vi "TestForceGraph 1.vi"() -> ()   [LabVIEW 2017]
panel:
  out "Signal Up":T1
  in  "FirstTouchAuto":T2={"FirstPeakforce"=2.0, "F_LengthView"=20, "A_LengthView "=10}
  in  "Auto":bool
  in  "FirstTouchDown":T2={"FirstPeakforce"=3.0, "F_LengthView"=20, "A_LengthView "=15}
  in  "ShowName":cluster{"ShowArrow":bool, "Alias":bool}
  in  "AngleMaxForce":bool=TRUE
  out "XY Up":cluster{"Y":dbl[], "Y":dbl[]}[](graph)
  in  "First Touch":bool
  in  "Path":path
  out "Filenames":string[](array[string])
  in  "FileType":string(combo)="DL"
  out "XY Down":cluster{"Y":dbl[], "Y":dbl[]}[](graph)
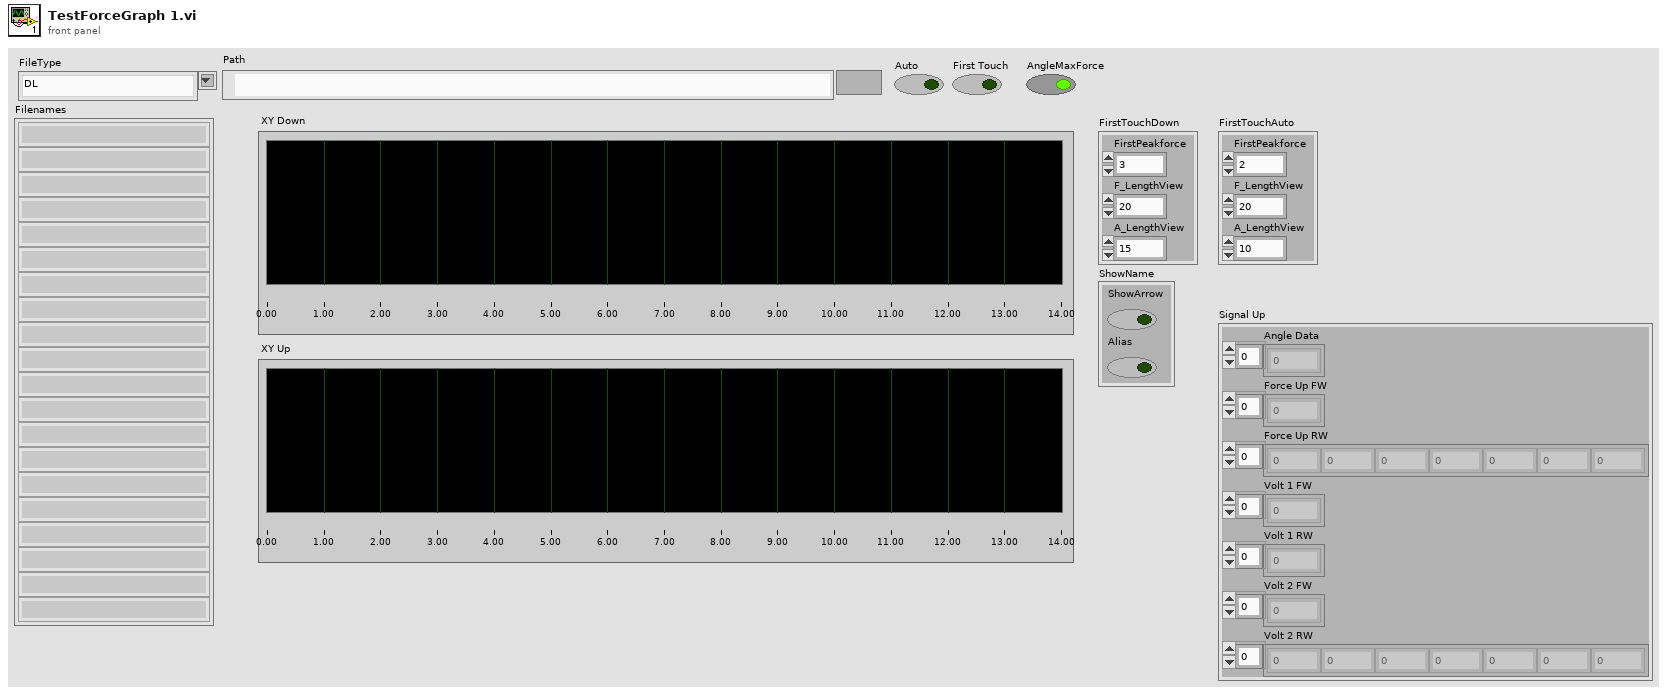
[diagram p1: front panel]
types:
  T1 = cluster{"Angle Data":dbl[], "Force Up FW":dbl[], "Force Up RW":dbl[], "Volt 1 FW":dbl[], "Volt 1 RW":dbl[], "Volt 2 FW":dbl[], "Volt 2 RW":dbl[]}
  T2 = cluster{"FirstPeakforce":dbl, "F_LengthView":i32, "A_LengthView ":i32}
  T3 = cluster{"DownMax":u16, "DownMin":u16, "UpMax":u16, "UpMin":u16}
  T4 = cluster{"Peak_Force":dbl, "Peak_Force_Tolerance":dbl, "Full_Angle":dbl, "Full_Angle_Tolerance":dbl, "ReturnForce":dbl}
  T5 = cluster{"Angle Data":dbl[], "Force Data":dbl[], "Volt Data 1":dbl[], "Volt Data 2":dbl[]}
  T6 = cluster{"Angle Data":dbl[], "Force Down FW":dbl[], "Force Down RW":dbl[], "Volt 1 FW":dbl[], "Volt 1 RW":dbl[], "Volt 2 FW":dbl[], "Volt 2 RW":dbl[]}
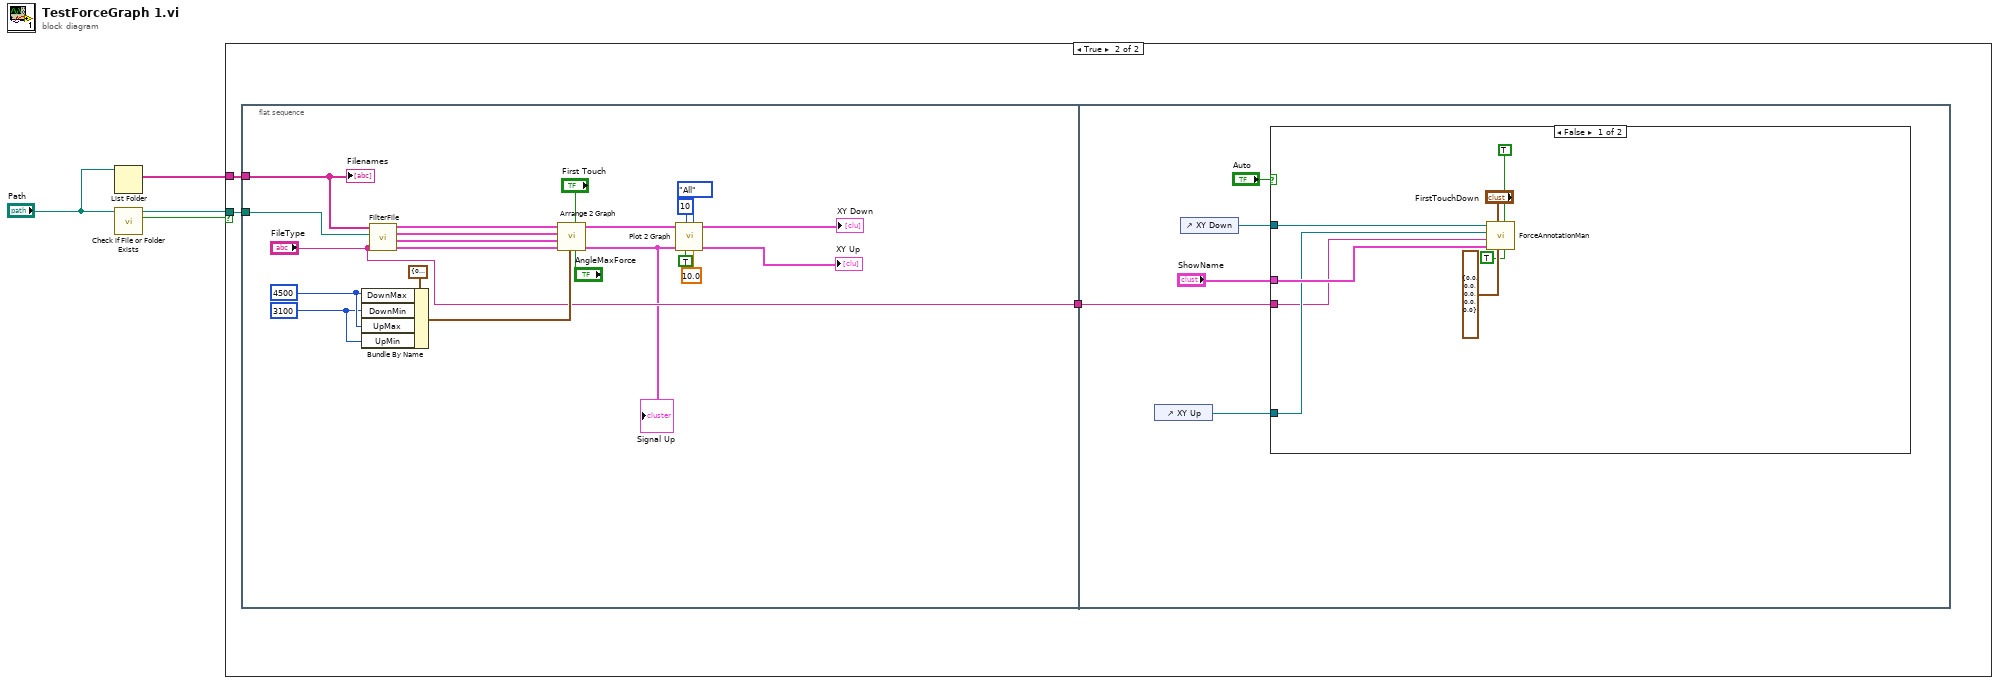
[diagram p0: block diagram]
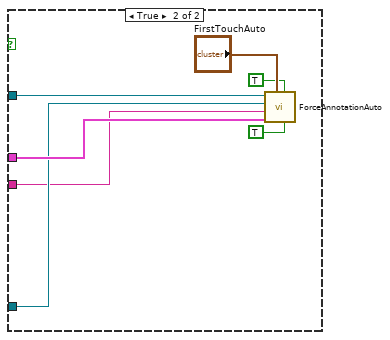
[diagram p3: hidden frame]
diagram:
  n1 = List Folder(path="Path") -> (filenames=w1:string[])  [unwired: 3 in, 3 out]
  n2 = call <vilib>:"Check if File or Folder Exists.vi"("path"="Path") -> ("file or folder exists?"=w4:bool, "dup path"=w2:path)  [unwired: 8 in, 1 out]
  n3 = case shown="True" w4 {
    tunnel: w2 -> [_ w7]
    tunnel: w1 -> [_ w5]
    frame False {
    }
    frame True {
      n4 = flat-sequence {
        tunnel: w7 -> [w22]
        tunnel: ["FileType"] -> w6
        tunnel: w5 -> [w18]
        tunnel: w6 -> [w33]
        frame #0 {
          w8 = u16 3100
          w9 = u16 4500
          n5 = Bundle By Name(cluster=T3 {"DownMax"=0, "DownMin"=0, "UpMax"=0, "UpMin"=0} ("AngleUpDown"), "DownMax"=w9, "DownMin"=w8, "UpMax"=w9, "UpMin"=w8) -> (w23:T3)
          n6 = call "FilterFile.vi"("FileType"="FileType", "Path"=w22, "Filenames"=w18) -> ("RW_Up"=w28:T5, "FW_Up"=w10:T5, "RW_Down"=w27:T5, "FW_Down"=w11:T5)  [unwired: 3 in, 2 out]
          n7 = call "Arrange 2 Graph.vi"("AngleMaxForce"="AngleMaxForce", "Find Fist Touch"="First Touch", "AngleUpDown"=w23, "Analog RW Up"=w28, "Analog FW Up"=w10, "Analog RW Down"=w27, "Analog FW Down"=w11) -> ("Signal Up"=w12:T1, "Signal Down"=w13:T6)  [unwired: 3 in]
          "Signal Up" <- w12
          n8 = call "Plot 2 Graph.vi"("VoltDevider"=10.0, "Type"=enum16{"All", "Force U+D", "Volt U+D"}."All", "EnableSmooth"=TRUE, "FillZeroFirstSignal"=10, "Analog Up"=w12, "Analog Down"=w13) -> ("XY Up"=→"XY Up":cluster{"Angle Data":dbl[], "Array":dbl[]}[], "XY Down"=→"XY Down":cluster{"Angle Data":dbl[], "Array":dbl[]}[])  [unwired: 4 in]
          "Filenames" <- w18
        }
        frame #1 {
          n9 = control-ref of="XY Up"() -> (w29:refnum<vi>)
          n10 = control-ref of="XY Down"() -> (w30:refnum<vi>)
          n11 = case shown="False" "Auto" {
            tunnel: w33 -> [w37 w44]
            tunnel: "ShowName" -> [w40 w46]
            tunnel: w30 -> [w39 w48]
            tunnel: w29 -> [w38 w45]
            frame False {
              n12 = call "ForceAnnotationMan.vi"("EnReturnForce"=TRUE, "EnFullAngle"=TRUE, "SpectConfig"=T4 {"Peak_Force"=0.0, "Peak_Force_Tolerance"=0.0, "Full_Angle"=0.0, "Full_Angle_Tolerance"=0.0, "ReturnForce"=0.0}, "FirstTouch"="FirstTouchDown", "ShowName"=w40, "Test Name"=w37, "Graph Up"=w38, "Graph Down"=w39) -> ()  [unwired: 4 out]
            }
            frame True {
              n13 = call "ForceAnnotationAuto.vi"("EnReturnForce"=TRUE, "EnFullAngle"=TRUE, "FirstTouch"="FirstTouchAuto", "ShowName"=w46, "Test Name"=w44, "Graph Up"=w45, "Graph Down"=w48) -> ()  [unwired: 1 in, 4 out]
            }
          }
        }
      }
    }
  }
